vi "Arrange VI Window.vi"(6 "Variant in":variant, 7 "Shift Pressed?":bool, 8 "error in (no error)":errorcluster, 10 "QD Combo Box Ref":refnum<vi>, 11 "QD Launch VI Ref":refnum<vi>) -> (0 "error out":errorcluster, 4 "Variant out":variant)   [LabVIEW 2012, in "Arrange VI Window.lvlib"]
doc: "When used on the front panel:\n-Arranges controls and indicators to be consistent with the connector pane arrangement. \n-Resizes and moves the front panel to a consistent top left location on the primary monitor.\n\nWhen used on the block diagram:\n-Scrolls the block diagram to a reasonable location relative to the top-most and/or left-most diagram object.\n-Resizes and moves the block diagram to a consistent top left location on the primary monitor.\n\nDefault Shortcut - [F]"
uses:
  Arrange VI Window.lvlib
panel:
  in  "Undo Name":string="Arrange VI Window"
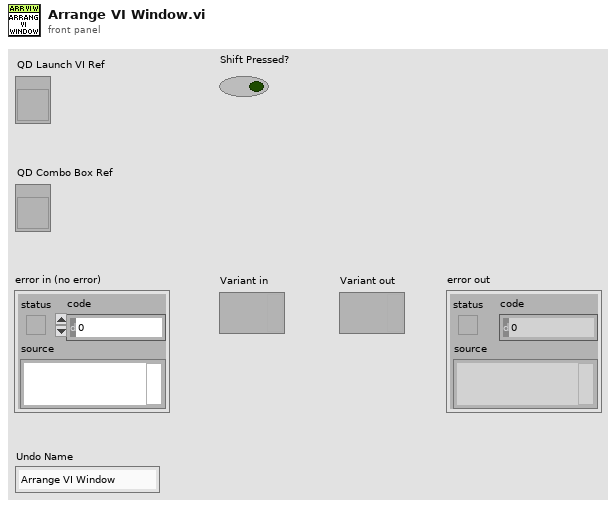
[diagram p1: front panel]
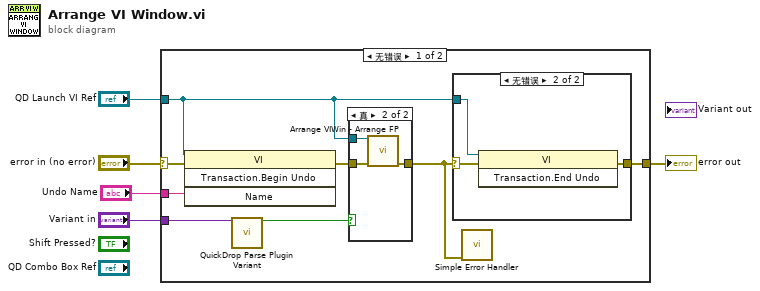
[diagram p0: block diagram]
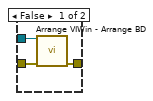
[diagram p2: hidden frame]
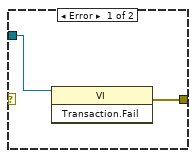
[diagram p3: hidden frame]
diagram:
  n1 = case shown="无错误" "error in (no error)" {
    selector: "error in (no error)" -> [w9 w25]
    tunnel: [w13 w25] -> w4
    tunnel: "QD Launch VI Ref" -> [w7 _]
    tunnel: "Variant in" -> [w12 _]
    tunnel: "Undo Name" -> [w6 _]
    frame No Error {
      n2 = invoke class="VI" method="Transaction.Begin Undo"(reference=w7, error in=w9, "Name"=w6) -> (error out=w8:errorcluster)  [unwired: 1 in, 3 out]
      n3 = call <vilib>:"QuickDrop Parse Plugin Variant.vi"("QDKS Variant in"=w12) -> ("QD Launch VI Panel?"=w11:bool)  [unwired: 12 in, 2 out]
      n4 = case shown="真" w11 {
        tunnel: w8 -> [w14 w18]
        tunnel: [w16 w19] -> w10
        tunnel: w7 -> [w15 w17]
        frame False {
          n5 = call "Arrange VIWin - Arrange BD.vi"("VI in"=w15, "error in"=w14) -> ("error out"=w16:errorcluster)  [unwired: 13 in]
        }
        frame True {
          n6 = call "Arrange VIWin - Arrange FP.vi"("VI in"=w17, "error in"=w18) -> ("error out"=w19:errorcluster)  [unwired: 13 in]
        }
      }
      n7 = case shown="无错误" w10 {
        selector: w10 -> [_ w22]
        tunnel: w7 -> [w20 w23]
        tunnel: [w21 w24] -> w13
        frame Error {
          n8 = invoke class="VI" method="Transaction.Fail"(reference=w20) -> (error out=w21:errorcluster)  [unwired: 2 in, 2 out]
        }
        frame No Error {
          n9 = invoke class="VI" method="Transaction.End Undo"(reference=w23, error in=w22) -> (error out=w24:errorcluster)  [unwired: 1 in, 2 out]
        }
      }
      n10 = call <vilib>:"Simple Error Handler.vi"("error in (no error)"=w10) -> ()  [unwired: 4 in, 5 out]
    }
    frame Error {
    }
  }
  "error out" <- w4
